vi "dynamic_signal_generation.vi"() -> ()   [LabVIEW 2020]
uses:
  <vilib>/DAQmx/write.llb/DAQmx Write (Analog Wfm 1Chan NSamp).vi
  <vilib>/DAQmx/create/channels.llb/DAQmx Create Channel (AO-Voltage-Basic).vi
  <vilib>/DAQmx/configure/timing.llb/DAQmx Timing (Sample Clock).vi
  <vilib>/Utility/file.llb/Read Delimited Spreadsheet (DBL).vi
  <vilib>/DAQmx/miscellaneous.llb/DAQmx Fill In Error Info.vi
  <resource>/objmgr/daqmx.rc
panel:
  in  "file to run":path=path "C:/Users/Puja/Desktop/Labview(PC)/Input_Signal/Sine_wave_data_without_time/data1_w1_NT_1per.txt"
  out "Input":waveform(dbl)(graph)
  in  "error in":errorcluster
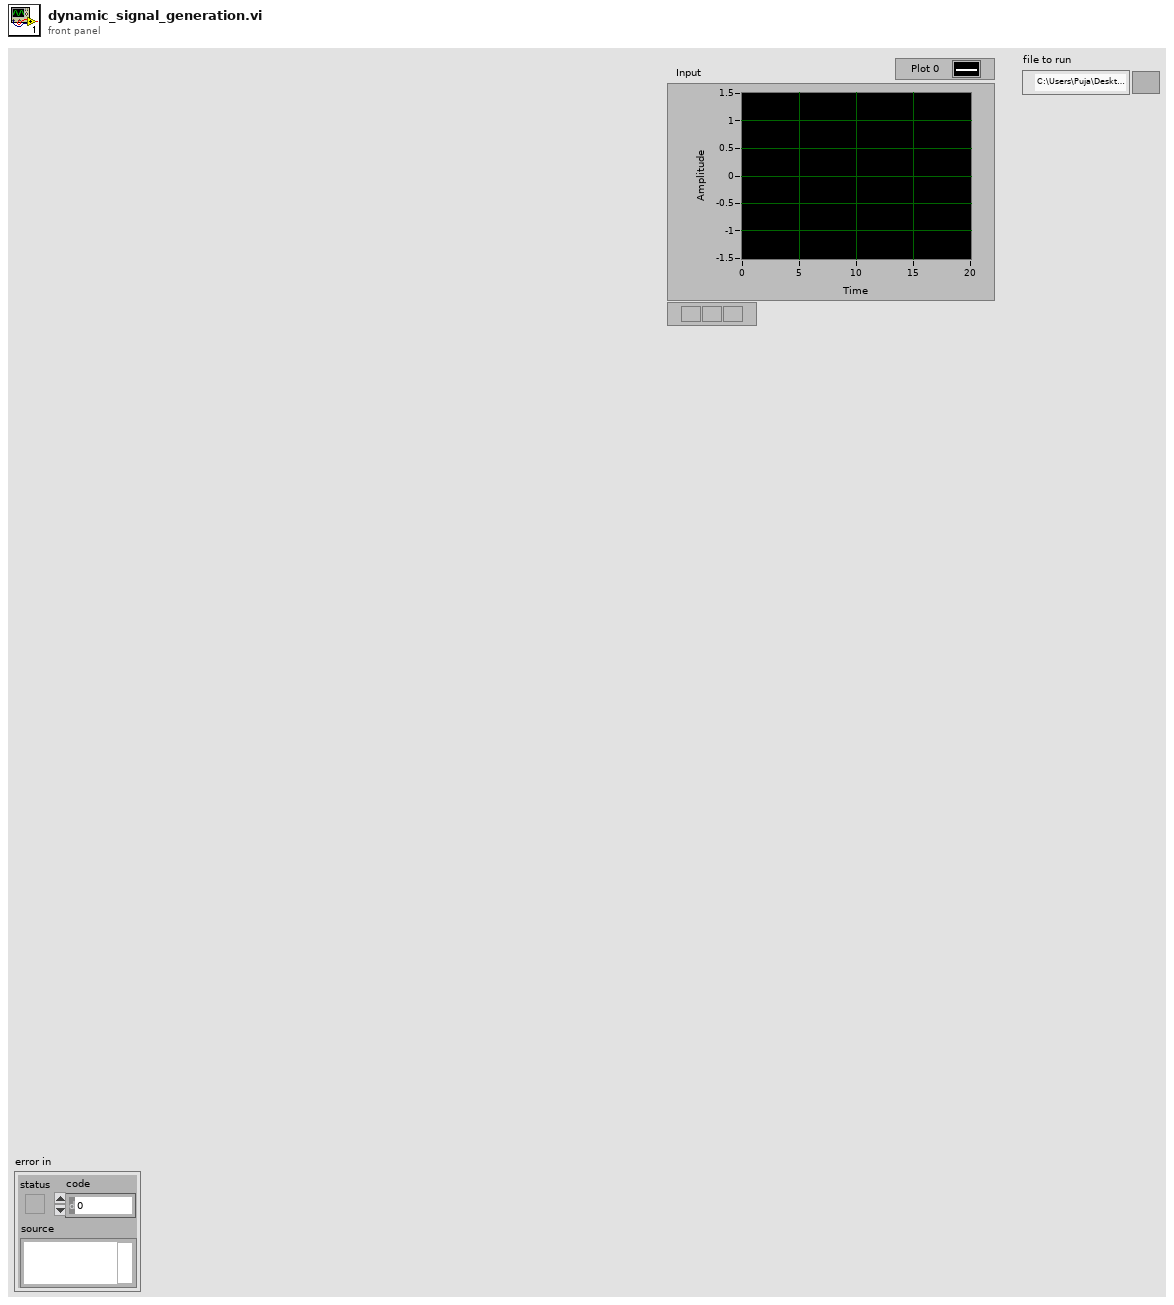
[diagram p1: front panel]
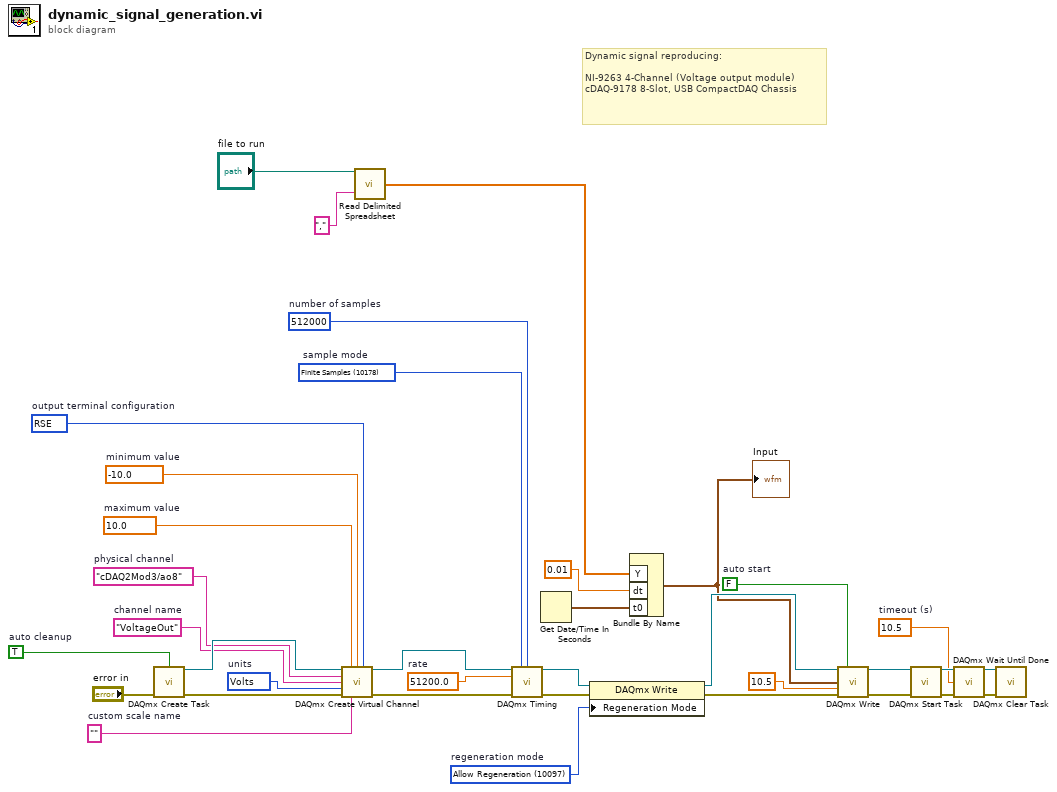
[diagram p0: block diagram]
diagram:
  w12 = 10097 items=["Allow Regeneration"=10097, "Do Not Allow Regeneration"=10158]  # regeneration mode
  w14 = 10178 items=["Finite Samples"=10178, "Continuous Samples"=10123, "Hardware Timed Single Point"=12522]  # sample mode
  w15 = 512000  # number of samples
  w16 = 51200.0  # rate
  w19 = 10083 items=["Default"=-1, "RSE"=10083, "Differential"=10106, "Pseudodifferential"=12529]  # output terminal configuration
  w20 = 10348 items=["Volts"=10348, "From Custom Scale"=10065]  # units
  w21 = "VoltageOut"  # channel name
  w23 = ""  # custom scale name
  w24 = -10.0  # minimum value
  w25 = 10.0  # maximum value
  w26 = "cDAQ2Mod3/ao8"  # physical channel
  w28 = TRUE  # auto cleanup
  w32 = 10.5  # timeout (s)
  w36 = FALSE  # auto start
  # "Dynamic signal reproducing:\n\nNI-9263 4-Channel (Voltage output module)\ncDAQ-9178 8-Slot, USB CompactDAQ Chassis"
  n1 = call <vilib>:"DAQmx Create Task.vi"("auto cleanup"=w28, "error in"="error in") -> ("task out"=w27:refnum<k21>, "error out"=w29:errorcluster)  [unwired: 12 in]
  n2 = call-poly <vilib>:"DAQmx Create Virtual Channel.vi"("task in"=w27, "maximum value"=w25, "minimum value"=w24, "output terminal configuration"=w19, "physical channels"=w26, "name to assign"=w21, "units"=w20, "error in"=w29, "custom scale name"=w23) -> ("task out"=w17:refnum<k21>, "error out"=w22:errorcluster)  [unwired: 5 in]
  n3 = call-poly <vilib>:"Read Delimited Spreadsheet.vi"("file path (dialog if empty)"="file to run", "delimiter (\\t)"=",") -> ("first row"=w5:dbl[])  [unwired: 8 in, 5 out]
  n4 = call-poly <vilib>:"DAQmx Timing.vi"("task/channels in"=w17, "sample mode"=w14, "samples per channel"=w15, "rate"=w16, "error in"=w22) -> ("task out"=w13:refnum<k21>, "error out"=w18:errorcluster)  [unwired: 9 in]
  n5 = Get Date/Time In Seconds() -> (seconds since 1Jan1904=w3:timestamp)
  n6 = property class="DAQmx Write"(reference=w13, error in=w18, "Regeneration Mode"=w12) -> (reference out=w11:refnum<k21>, error out=w10:errorcluster)
  n7 = Bundle By Name("Y"=w5, "dt"=0.01, "t0"=w3) -> (w1:waveform(dbl))  [unwired: 1 in]
  "Input" <- w1
  n8 = call-poly <vilib>:"DAQmx Write.vi"("task/channels in"=w11, "auto start"=w36, "data"=w1, "timeout"=10.5, "error in"=w10) -> ("task out"=w8:refnum<k21>, "error out"=w7:errorcluster)  [unwired: 8 in, 1 out]
  n9 = call <vilib>:"DAQmx Start Task.vi"("task/channels in"=w8, "error in"=w7) -> ("task out"=w35:refnum<k21>, "error out"=w34:errorcluster)  [unwired: 12 in]
  n10 = call <vilib>:"DAQmx Wait Until Done.vi"("task/channels in"=w35, "timeout (sec)"=w32, "error in"=w34) -> ("task out"=w31:refnum<k21>, "error out"=w33:errorcluster)  [unwired: 11 in]
  n11 = call <vilib>:"DAQmx Clear Task.vi"("task in"=w31, "error in"=w33) -> ()  [unwired: 13 in, 1 out]
